vi "Interfaz_Usuario.vi"() -> ()   [LabVIEW 2014]
uses:
  <vilib>/Utility/file.llb/Read From Spreadsheet File (DBL).vi
panel:
  out "Tamaño de la data":i32[](array[numeric])
  out "first row":dbl[](array[numeric]) format="%0.3f"
  out "all rows":dbl[][](array[numeric]) format="%0.3f"
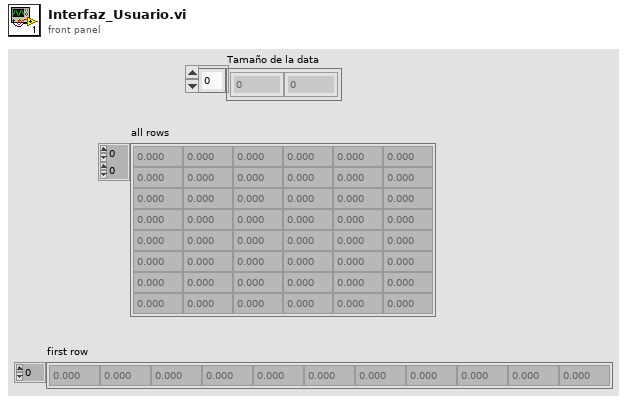
[diagram p1: front panel]
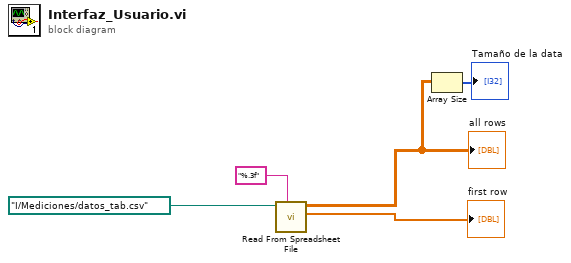
[diagram p0: block diagram]
diagram:
  n1 = call-poly <vilib>:"Read From Spreadsheet File.vi"("format (%.3f)"="%.3f", "file path (dialog if empty)"=path "I:/Mediciones/datos_tab.csv") -> ("first row"=→"first row":dbl[], "all rows"=w3:dbl[][])  [unwired: 5 in, 3 out]
  "all rows" <- w3
  n2 = Array Size(array=w3) -> (size(s)=→"Tamaño de la data":i32[])
